vi "Read Buffer Data.vi"(0 "VISA resource name":refnum<visa-resource-name>, 1 "Zero Time Axis (T)":bool=TRUE, 11 "error in (no error)":errorcluster) -> (4 "VISA resource name out":refnum<visa-resource-name>, 6 "Instrument Buffer Data":cluster{dbl[], dbl[]}(graph), 15 "error out":errorcluster)   [LabVIEW 2024, in "Keithley 648X Series.lvlib"]
doc: "Reads the reading data stored in the data buffer as an XY plot based on reading value and time.\n\n<b>Note:</b>\nThe buffer must have data before reading, ot the instrument will return data stale error."
uses:
  <instrlib>/Keithley 648X Series/Keithley 648X Series.lvlib
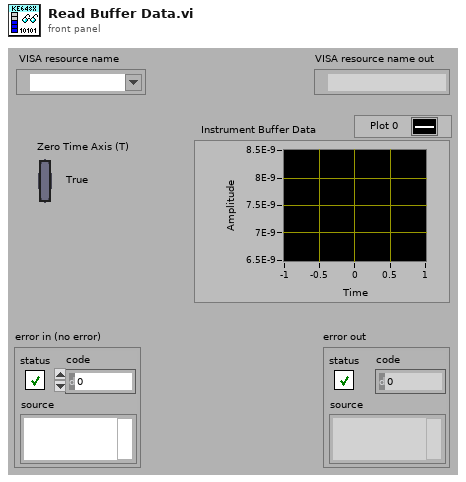
[diagram p1: front panel]
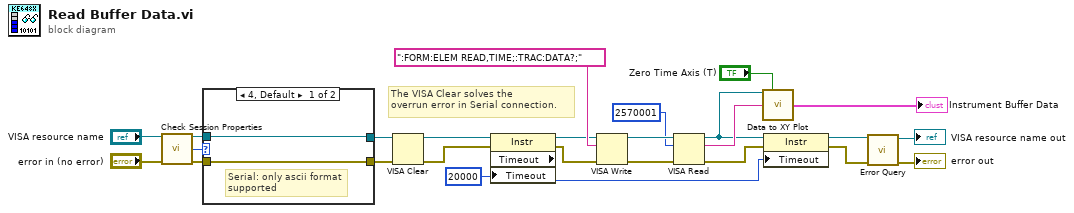
[diagram p0: block diagram]
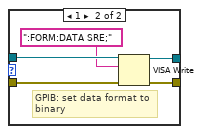
[diagram p2: hidden frame]
diagram:
  # "The VISA Clear solves the\noverrun error in Serial connection."
  n1 = call <instrlib>:"Check Session Properties.vi"("VISA resource name"="VISA resource name", "error in (no error)"="error in (no error)") -> ("VISA resource name out"=w17:refnum<visa-resource-name>, "Interface Type"=w18:u16, "error out"=w19:errorcluster)  [unwired: 10 in, 1 out]
  n2 = case shown="4, Default" w18 {
    tunnel: [w27 w32] -> w5
    tunnel: [w26 w31] -> w2
    tunnel: w19 -> [w26 w30]
    tunnel: w17 -> [w27 w29]
    frame 4, Default {
      # "Serial: only ascii format\nsupported"
    }
    frame 1 {
      # "GPIB: set data format to\nbinary"
      n3 = VISA Write(VISA resource name=w29, write buffer=":FORM:DATA SRE;", error in (no error)=w30) -> (VISA resource name out=w32:refnum<visa-resource-name>, error out=w31:errorcluster)  [unwired: 1 out]
    }
  }
  n4 = VISA Clear(VISA resource name=w5, error in (no error)=w2) -> (VISA resource name out=w4:refnum<visa-resource-name>)  [unwired: 1 out]
  n5 = property class="Instr"(reference=w4, error in=w2, "Timeout"=u32 20000 ("General Settings:Timeout Value")) -> (reference out=w3:refnum<visa-resource-name>, error out=w1:errorcluster, "Timeout"=w7:u32)
  n6 = VISA Write(VISA resource name=w3, write buffer=":FORM:ELEM READ,TIME;:TRAC:DATA?;" ("Initiate"), error in (no error)=w1) -> (VISA resource name out=w24:refnum<visa-resource-name>, error out=w23:errorcluster)  [unwired: 1 out]
  n7 = VISA Read(VISA resource name=w24, byte count=u32 2570001, error in (no error)=w23) -> (VISA resource name out=w11:refnum<visa-resource-name>, read buffer=w13:string, error out=w9:errorcluster)  [unwired: 1 out]
  n8 = call <instrlib>:"Data to XY Plot.vi"("VISA resource name"=w11, "Zero Time Axis (T)"="Zero Time Axis (T)", "String of Data"=w13) -> ("XY Graph"=→"Instrument Buffer Data":cluster{dbl[], dbl[]})  [unwired: 12 in]
  n9 = property class="Instr"(reference=w11, error in=w9, "Timeout"=w7) -> (reference out=w10:refnum<visa-resource-name>, error out=w8:errorcluster)
  n10 = call <instrlib>:"Error Query.vi"("error in (no error)"=w8, "VISA resource name"=w10) -> ("error out"=→"error out":errorcluster, "VISA resource name out"=→"VISA resource name out":refnum<visa-resource-name>)  [unwired: 6 in, 2 out]
